vi "Load VI.vi"(8 "error in (no error)":errorcluster, 11 "vi path":path) -> (0 "error out":errorcluster, 3 "VI out":refnum<vi>)   [LabVIEW 2025, in "Tools.lvlib"]
uses:
  Tools/Tools.lvlib
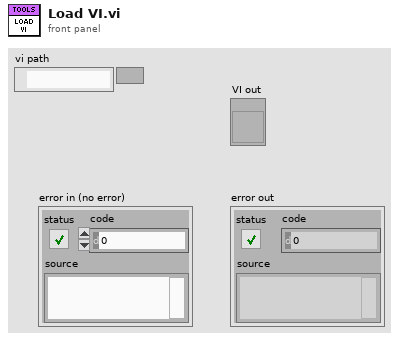
[diagram p1: front panel]
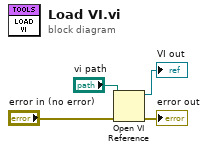
[diagram p0: block diagram]
diagram:
  n1 = Open VI Reference(vi path="vi path", error in (no error)="error in (no error)") -> (vi reference=→"VI out":refnum<vi>, error out=→"error out":errorcluster)  [unwired: 4 in]
